vi "PC_Daten zu cRIO.vi"   [LabVIEW 2020, in "Kommunikation mit cRIO.lvlib"]
uses:
  Kommunikation mit cRIO.lvlib
  Bildwechsel/Bild-Auswahl.ctl
  Aktionen FGV Druckregler.ctl
  Funktionstasten/Funktionstasten-Aktion.ctl
  Seiten/Gaszuordnung AO/ANA-OUT Aktionen.ctl
  Seiten/Erweiterte Konfig/FGV PID Aktionen.ctl
  Stoerungen/FGV Stoerung aufnehmen Aktion.ctl
  Seiten/Erweiterte Konfig/Aktionen LN2 Dewar Spuelen.ctl
  EPA 1065/Dichtheitstest 1065-345/Aktion Leak Daten.ctl
  Funktionstasten/FGV Erweiterte Bedienung Aktion.ctl
  Seiten/CalGas Aufschaltung/FGV CalGas Aktionen.ctl
  Auto Kalibrieren/Aktion FGV CalZustand.ctl
  Status Analysatoren/Aktion Status Analysatoren.ctl
  Seiten/System Einstellungen V2/Aktioen FGV System.ctl
  Seiten/System Einstellungen V2/Aktioen FGV System Konstanten.ctl
  Auto Kalibrieren/Aktion FGV Autokal GT.ctl
  Seiten/Anlagengrenzwerte/Aktion Durchflussaenderung.ctl
  Allgemein/Aktion FGV Aufheizphase.ctl
  EPA 1065/T90 1065-308/Aktion FGV T90.ctl
  Seiten/Anlagenuebersicht/VisBx Anzeige/Aktion FGV Ventile manuell schalten Crio.ctl
  Allgemein/Aktionen Daten am cRIO speichern.ctl
  Seiten/Anlagengrenzwerte/FGV Anlagengrenzwerte Aktionen.ctl
  Seiten/CAN Konfig/Aktion FGV CAN.ctl
  Seiten/Anlagengrenzwerte/Anlagengrenzwerte.lvlib
  Seiten/Erweiterte Konfig/Erweiterte Konfig.lvlib
  Bildwechsel/Bildwechsel.lvlib
  Allgemein/allgemeine Sub-VIs.lvlib
  Funktionstasten/Funktionstasten.lvlib
  Seiten/Gaszuordnung AO/Gaszuordnung AO.lvlib
  Stoerungen/Stoerungen.lvlib
  Seiten/System Einstellungen V2/System Einstellungen V2.lvlib
  EPA 1065/Dichtheitstest 1065-345/Dichtheitstest 1065-345.lvlib
  Auto Kalibrieren/Auto Kalibrieren.lvlib
  Seiten/CalGas Aufschaltung/CalGas Aufschaltung.lvlib
  Status Analysatoren/Status Analysatoren.lvlib
  EPA 1065/T90 1065-308/T90 Test 1065-308.lvlib
  Seiten/Anlagenuebersicht/VisBx Anzeige/Anlagenuebersicht.lvlib
  Seiten/CAN Konfig/CAN Konfig.lvlib
types:
  T1 = typedef "Anlagenuebersicht.lvlib/Aktion FGV Ventile manuell schalten Crio.ctl" = enum16{"lesen", "Ventile schalten", "Testbetrieb aktiv", "Testbetrieb inaktiv", "Anzeige Ventilstellung"}
  T2 = typedef "EPA 1065.lvlib/T90 Test 1065-308.lvlib/Aktion FGV T90.ctl" = enum16{"lesen", "Konfig Daten", "speichern", "laden", "T90 aktiv", "T90 inaktiv", "Ext. Ventil aktivieren", "Ext. Ventil deaktivieren", "N2 spülen aktiv", "N2 spülen inaktiv", "Ergebnis Textfile"}
  T3 = typedef "allgemeine Sub-VIs.lvlib/Aktion FGV Aufheizphase.ctl" = enum16{"init", "lesen", "PNS Filterblock", "PNS HL1", "PNS HL2", "PNS HL3", "PNS HL4", "FTIR Messzelle", "HL 1", "HL 2", "HL zu FTIR", "auswerten"}
  T4 = typedef "Bildwechsel.lvlib/Bild-Auswahl.ctl" = enum16{"lesen", "Initialisieren", "Beenden", "Grafik", "Anlagenübersicht", "Anlagengrenzwerte", "Log Konfig", "Gaszuordnung AO", "Erw. Konfiguration", "FT-IR  ", "Störmeldungen", "Störmeldepuffer", "Störmeldekonfig", "PNS Grenzwerte", "Statusübersicht", "Linearisierung", "ARN", "EPA Dichtheitstest", "FID", "PMA", "CalGas", "Lambda", "Interference", "Amium PNS", "EPA T90", "Interference N2O", "Scheduler", "Systemeinstellungen", "EPA Drift", "CAN Konfig"}
  T5 = typedef "Anlagengrenzwerte.lvlib/Aktion Durchflussaenderung.ctl" = enum16{"lesen", "Statusänderung", "Reset"}
  T6 = typedef "Auto Kalibrieren.lvlib/Aktion FGV Autokal GT.ctl" = enum16{"lesen", "Autokal GT", "Referenz Start"}
  T7 = typedef "System Einstellungen V2.lvlib/Aktioen FGV System Konstanten.ctl" = enum16{"lesen", "laden", "speichern", "Sprache"}
  T8 = typedef "System Einstellungen V2.lvlib/Aktioen FGV System.ctl" = enum16{"lesen", "laden", "speichern", "Optionen schreiben", "Zeitstempel", "Reset BMP", "Reset SQP", "Wartung", "Werkseinstellung"}
  T9 = typedef "Status Analysatoren.lvlib/Aktion Status Analysatoren.ctl" = enum16{"lesen", "initialisieren", "Analysatoren aktiv", "FTIR Fehler", "FID Fehler", "PMA Fehler", "Felder einfärben"}
  T10 = typedef "Auto Kalibrieren.lvlib/Aktion FGV CalZustand.ctl" = enum16{"lesen", "Cal FTIR", "Cal FID CH4", "Cal PMA", "init", "Cal FID THC", "THC CG Eingang"}
  T11 = typedef "CalGas Aufschaltung.lvlib/FGV CalGas Aktionen.ctl" = enum16{"lesen", "Analysator Auswahl", "Def.CalGas", "Aufschaltung CalGas", "laden", "speichern", "KAL extrahieren"}
  T12 = typedef "Funktionstasten.lvlib/FGV Erweiterte Bedienung Aktion.ctl" = enum16{"Lesen", "Initialisieren", "N2 zu PNS", "Chart wechsel"}
  T13 = typedef "EPA 1065.lvlib/Dichtheitstest 1065-345.lvlib/Aktion Leak Daten.ctl" = enum16{"lesen", "laden", "speichern", "Volumen", "berechnen", "Leak check aktiv", "Leak Zustand", "Pfad", "Pfad speichern"}
  T14 = typedef "Erweiterte Konfig.lvlib/Aktionen LN2 Dewar Spuelen.ctl" = enum16{"lesen", "schreiben", "prüfen"}
  T15 = typedef "Stoerungen.lvlib/FGV Stoerung aufnehmen Aktion.ctl" = enum16{"Initialisieren", "Schreiben", "Lesen", "Quittieren", "quit. löschen"}
  T16 = typedef "Erweiterte Konfig.lvlib/FGV PID Aktionen.ctl" = enum16{"Lesen", "Schreiben PID", "Schreiben Sonstige", "Dichtheitstest", "Aktionen Dicht.", "Parameter Sensor"}
  T17 = typedef "Gaszuordnung AO.lvlib/ANA-OUT Aktionen.ctl" = enum16{"lesen", "Gase schreiben"}
  T18 = typedef "Funktionstasten.lvlib/Funktionstasten-Aktion.ctl" = enum16{"Initialisieren", "Zustand setzen", "Taste gedrückt", "Fehler speichern", "Lesen", "Manuell", "Remote", "Bitparallel", "Samplepoint", "Zeit Prüfen", "reset Umschalten"}
  T19 = typedef "Kommunikation mit cRIO.lvlib/Aktionen FGV Druckregler.ctl" = enum16{"lesen", "Parameter", "Istwerte", "laden", "speichern"}
  T20 = typedef "Status Analysatoren.lvlib/Status.ctl" = cluster{"FT-IR aktiv":bool, "FT-IR Fehler":bool, "FID aktiv":bool, "FID Fehler":bool, "PMA aktiv":bool, "PMA Fehler":bool}
  T21 = typedef "Erweiterte Konfig.lvlib/Aktionen Dichtheitstest.ctl" = enum16{"Initialisieren", "Unterdruck aufbauen", "Prop schließen", "Warten", "Auswertung", "Fertig"}
  T22 = typedef "System Einstellungen V2.lvlib/Optionen.ctl" = cluster{"Störmeldep.":bool, "Betriebszustände":bool, "AK in ppm":bool, "log Cal-Gas":bool, "log 0-Gas":bool, "Durchflusssensor 0-5V":bool, "PNS?":bool, "Mit N2 spülen":bool, "TRE08":bool, "Amium 10-Fach":bool, "Verticale Scrollbar aktiv":bool, "Loggingtakt":bool, "AK Rezeptwechsel gleich wie MKS":bool, "NG ECO":bool}
  T23 = typedef "EPA 1065.lvlib/Dichtheitstest 1065-345.lvlib/Aktion Leak check durchfuehren.ctl" = enum16{"initialisieren", "Unterdruck erzeugen", "Ventile schließen", "Warten", "Auswertung", "fertig", "PDF erstellen", "abbrechen"}
  T24 = typedef "CalGas Aufschaltung.lvlib/Aufschaltung CalGas.ctl" = cluster{"Kalibriergas":T25, "Aufschaltpunkt":T26, "Analysator":T27}
  T25 = typedef "Auswahlfeld.ctl" = u16
  T26 = typedef "CalGas Aufschaltung.lvlib/Auswahl Aufschaltpunkt.ctl" = enum16{"über Filterblock", "Analysator direkt", "über PNS", "Entnahme", "Gasdivider"}
  T27 = typedef "CalGas Aufschaltung.lvlib/Auswahl Analysator.ctl" = enum16{"FT-IR", "FID", "PMA", "PMA/FID/FT-IR"}
  T28 = typedef "allgemeine Sub-VIs.lvlib/Aktionen Daten am cRIO speichern.ctl" = enum16{"lesen", "speichern setzen", "speichern reset", "gespeichert"}
  T29 = typedef "Anlagengrenzwerte.lvlib/FGV Anlagengrenzwerte Aktionen.ctl" = enum16{"Lesen", "Grenzwerte schreiben"}
  T30 = typedef "CAN Konfig.lvlib/Aktion FGV CAN.ctl" = enum16{"lesen", "schreiben Konfig", "Status", "Messdaten", "laden", "speichern", "CAN Data"}
  T31 = typedef "Anlagengrenzwerte.lvlib/Anlagen-Grenzwerte Anzeige.ctl" = cluster{"Eingangsdruck FT-IR:":T32, "Durchfluss FT-IR:":T32, "Durchfluss CalGas:":T32, "Druck Ausgang:":T32, "Druck Kalter Block:":T32, "Heizleitungen intern:":T32, "Heizleitung zu FT-IR:":T32, "Heizung Filterblock:":T32, "Heizung Pumpe:":T32, "Heizleitung Extern SP1:":T32, "Heizleitung Extern SP2:":T32, "FT-IR Heizung Messzelle:":T32, "Schaltschranktemperatur:":T32, "Gaskühler:":T32}
  T32 = typedef "Anlagengrenzwerte.lvlib/Anlagen-Parameter Anzeige.ctl" = cluster{"Sollwert":sgl, "Warn-Min":sgl, "Warn-Max":sgl, "Abschalt-Min":sgl, "Abschalt-Max":sgl, "Regler":u16}
  T33 = cluster{"Sollwert":sgl, "Warn-Min":sgl, "Warn-Max":sgl, "Abschalt-Min":sgl, "Abschalt-Max":sgl, "Regler":sgl}
  T34 = typedef "Erweiterte Konfig.lvlib/Sonstige Parameter.ctl" = cluster{"Lüfter langsam":sgl, "Lüfter schnell":sgl, "FT-IR Kühlung Soll":sgl, "FT-IR Kühlung Max":sgl, "Überwachung":T25, "Befüllung aktiv":T35, "Stickstoff Befüllzeit":sgl, "Befüllintervall":sgl, "Kalibrierwert FT-IR":sgl, "Offset Ausgang":sgl, "Offset FT-IR":sgl, "Offset Druck FT-IR":sgl, "Dichtheitstest Zeit":sgl, "Dichtheitstest Abfall":sgl, "Dichtheitstest Umfang":T36, "Offset Umgebung":sgl, "Max Taupunkt":sgl, "Pumpendrehzahl":sgl, "ext. Befüllung":T35, "Ext. Stickstoff Befüllzeit":sgl}
  T35 = typedef "LogKonfig.lvlib/Auswahlfeld aktiviert-deaktiviert.ctl" = u16
  T36 = typedef "Erweiterte Konfig.lvlib/Dichtheitstest Umfang.ctl" = u16
  T37 = typedef "Erweiterte Konfig.lvlib/PID-Parameter Anzeige.ctl" = cluster{"Heizung\nFilterblock":T38, "Heizung\nPumpe":T38, "Heizung\nHeizleitungen":T38, "Heizleitung\nExtern":T38, "Heizung\nFB-Druckregler":T38}
  T38 = typedef "Erweiterte Konfig.lvlib/PID-Parameter.ctl" = cluster{"P-Anteil":T39, "I-Anteil":T39, "D-Anteil":T39, "Regelzonengr.":T39, "max. OUT":T39}
  T39 = typedef "Zahlen-Eingabefeld.ctl" = sgl
  T40 = typedef "Erweiterte Konfig.lvlib/Parameter Sensoren.ctl" = cluster{"Kal.Durchfl.FTIR":sgl, "Kal.Durchfl.PMA":sgl, "Offset Durchfl.FTIR":sgl, "Offset Druck Ausgang":sgl, "Offset Druck Umgebung":sgl, "Offset Durchfl.PMA":sgl, "Offset Druck CG PMA":sgl, "Offset Druck CG":sgl, "Offset Druck FTIR IAG":sgl, "Druck Kalter Block":sgl}
  T41 = cluster{"Lüfter langsam":sgl, "Lüfter schnell":sgl, "FT-IR Kühlung Soll":sgl, "FT-IR Kühlung Max":sgl, sgl, sgl, "Stickstoff Befüllzeit":sgl, "Befüllintervall":sgl, "Kalibrierwert FT-IR":sgl, "Offset Ausgang":sgl, "Offset FT-IR":sgl, "Offset Druck FT-IR":sgl, "Dichtheitstest Zeit":sgl, "Dichtheitstest Abfall":sgl, sgl, "Offset Umgebung":sgl, "Max Taupunkt":sgl, "Pumpendrehzahl":sgl, sgl, "Ext. Stickstoff Befüllzeit":sgl}
  T42 = typedef "CAN Konfig.lvlib/Konfig Daten PC.ctl" = cluster{"Baude Rate":T43, "COM state":u8, "Frame-ID FTIR Start":u32, "Frame-ID FTIR End":u32, "Frame-ID Status Start":u32, "Frame-ID Status End":u32, "Zustand Information":u32, "Aktion":u32, "Frame-ID FTIR Arry":u32[], "Frame-ID Status Arry":u32[], "GPS Start":u32, "Interface":refnum<k21>}
  T43 = typedef "CAN Interface.lvlib/Baude Rate.ctl" = u32
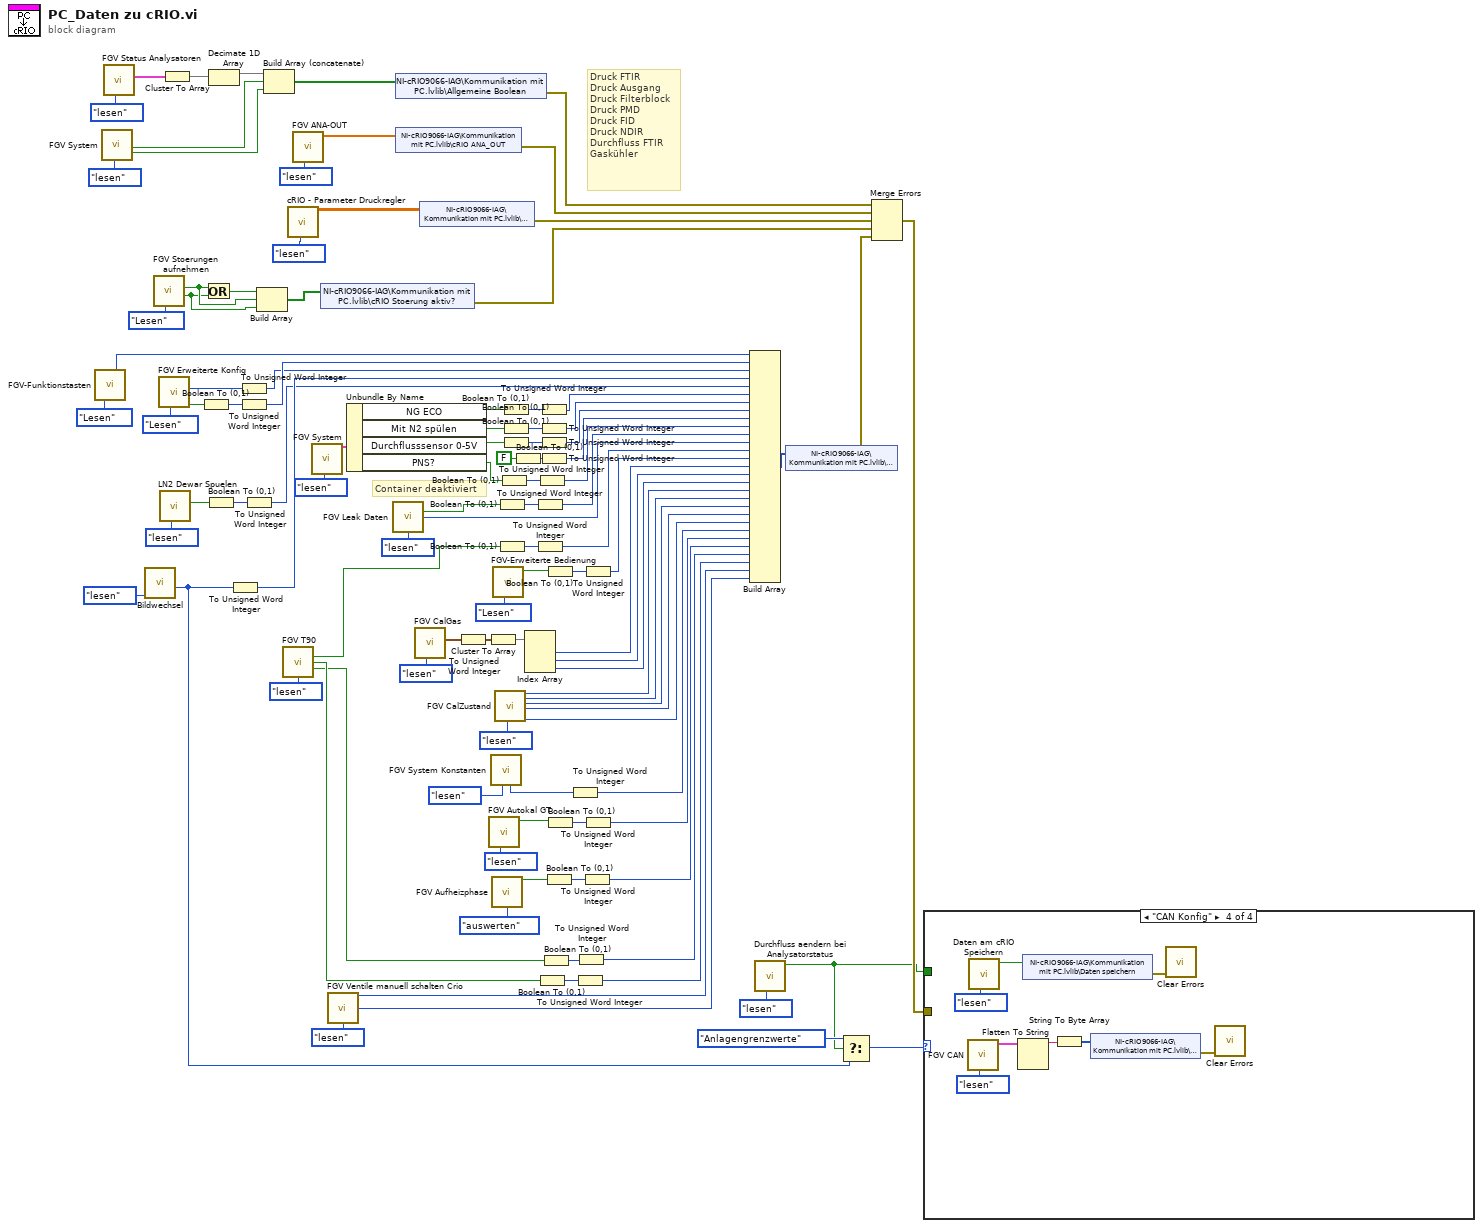
[diagram p0: block diagram]
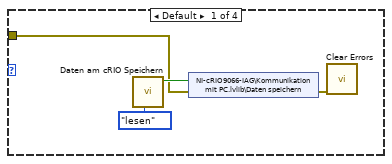
[diagram p2: hidden frame]
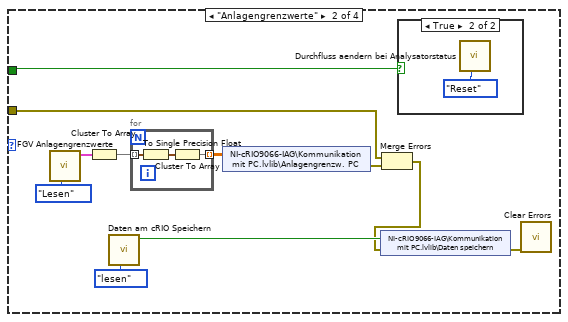
[diagram p3: hidden frame]
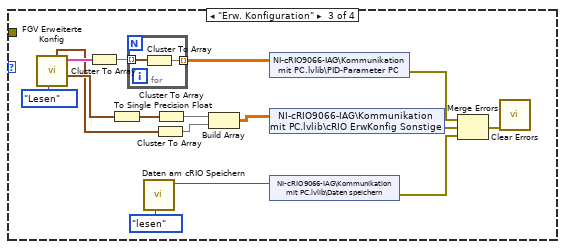
[diagram p5: hidden frame]
diagram:
  # "Container deaktiviert"
  # "Druck FTIR\nDruck Ausgang\nDruck Filterblock\nDruck PMD\nDruck FID\nDruck NDIR\nDurchfluss FTIR\nGaskühler"
  n1 = call "FGV-Funktionstasten.vi"("Aktion"=Funktionstasten-Aktion."Lesen") -> ("Samplepoint"=w101:u16)  [unwired: 7 in, 7 out]
  n2 = call "FGV System.vi"("Aktionen"=Aktioen_FGV_System."lesen") -> ("Reset BMP"=w36:bool, "Reset SQP"=w35:bool)  [unwired: 12 in, 5 out]
  n3 = call "FGV Status Analysatoren.vi"("Aktionen"=Aktion_Status_Analysatoren."lesen") -> ("Status Analysatoren"=w41:T20)  [unwired: 10 in]
  n4 = call "Bildwechsel.vi"("nächstes Bild"=Bild-Auswahl."lesen") -> ("aktuelle Bildnummer"=w23:T4)  [unwired: 9 in, 1 out]
  n5 = call "FGV Stoerungen aufnehmen.vi"("FGV Störung aufnehmen Aktion"=FGV_Stoerung_aufnehmen_Aktion."Lesen") -> ("abschalten"=w14:bool, "warnen"=w15:bool)  [unwired: 7 in, 2 out]
  n6 = call "FGV Erweiterte Konfig.vi"("Aktion"=FGV_PID_Aktionen."Lesen") -> ("Dichtheitstest?"=w98:bool, "Aktionen Dichtheitstest"=w99:T21)  [unwired: 6 in, 3 out]
  n7 = call "LN2 Dewar Spuelen.vi"("Aktionen"=Aktionen_LN2_Dewar_Spuelen."lesen") -> ("LN2 Spülen?"=w83:bool)  [unwired: 10 in]
  n8 = Cluster To Array(cluster=w41) -> (array=w40:bool[])
  n9 = Boolean To (0,1)(Boolean=w98) -> (0, 1=w100:i16)
  n10 = Or(x=w15, y=w14) -> (x .or. y?=w86:bool)
  n11 = Boolean To (0,1)(Boolean=w83) -> (0, 1=w84:i16)
  n12 = Decimate 1D Array(w40) -> (w39:bool[])  [unwired: 1 out]
  n13 = To Unsigned Word Integer(number=w23) -> (unsigned 16bit integer=w95:u16)
  n14 = To Unsigned Word Integer(number=w99) -> (unsigned 16bit integer=w96:u16)
  n15 = To Unsigned Word Integer(number=w100) -> (unsigned 16bit integer=w97:u16)
  n16 = To Unsigned Word Integer(number=w84) -> (unsigned 16bit integer=w82:u16)
  n17 = Build Array(w86, w15, w14) -> (w16:bool[])
  n18 = Build Array (concatenate)(w39, w36, w35) -> (w38:bool[])
  n19 = call "FGV T90.vi"("Aktion"=Aktion_FGV_T90."lesen") -> ("T90 Aktiv"=w10:bool, "Ext. Ventil aktiv"=w8:bool, "N2 spülen aktiv"=w7:bool)  [unwired: 9 in, 3 out]
  n20 = call "cRIO - Parameter Druckregler.vi"("Aktion"=Aktionen_FGV_Druckregler."lesen") -> ("Parameter Regler"=w93:sgl[][])  [unwired: 9 in, 9 out]
  n21 = call "FGV ANA-OUT.vi"("Aktion"=ANA-OUT_Aktionen."lesen") -> ("ANA-OUT 1-16"=w91:sgl[])  [unwired: 10 in]
  n22 = call "FGV System.vi"("Aktionen"=Aktioen_FGV_System."lesen") -> ("Optionen"=w80:T22)  [unwired: 12 in, 6 out]
  n23 = shared-variable "NI-cRIO9066-IAG\\Kommunikation mit PC.lvlib\\cRIO Stoerung aktiv?"(w16) -> (error out=w94:errorcluster)  [unwired: 1 in]
  n24 = call "FGV Ventile manuell schalten Crio.vi"("Aktion"=Aktion_FGV_Ventile_manuell_schalten_Crio."lesen") -> ("Ventile schalten"=w2:u32, "Betrieb"=w1:u16)  [unwired: 11 in, 2 out]
  n25 = Unbundle By Name(w80) -> ("NG ECO"=w4:bool, "Mit N2 spülen"=w76:bool, "Durchflusssensor 0-5V"=w73:bool, "PNS?"=w69:bool)
  n26 = call "FGV Leak Daten.vi"("Aktion"=Aktion_Leak_Daten."lesen") -> ("Dichtheitstest aktiv"=w65:bool, "Dichtheitstest Zustand"=w63:T23)  [unwired: 10 in, 3 out]
  n27 = shared-variable "NI-cRIO9066-IAG\\Kommunikation mit PC.lvlib\\Allgemeine Boolean"(w38) -> (error out=w43:errorcluster)  [unwired: 1 in]
  n28 = shared-variable "NI-cRIO9066-IAG\\Kommunikation mit PC.lvlib\\cRIO ANA_OUT"(w91) -> (error out=w90:errorcluster)  [unwired: 1 in]
  n29 = call "FGV CalGas.vi"("Aktionen"=FGV_CalGas_Aktionen."lesen") -> ("Aufschaltung CalGas"=w53:T24)  [unwired: 6 in, 4 out]
  n30 = shared-variable "NI-cRIO9066-IAG\\Kommunikation mit PC.lvlib\\Param.Regler"(w93) -> (error out=w92:errorcluster)  [unwired: 1 in]
  n31 = To Unsigned Word Integer(number=w53) -> (unsigned 16bit integer=w52:cluster{"Kalibriergas":T25, u16, u16})
  n32 = Cluster To Array(cluster=w52) -> (array=w51:T25[])
  n33 = call "FGV Autokal GT.vi"("Aktion FGV AutoKal"=Aktion_FGV_Autokal_GT."lesen") -> ("Autokal GT Aktiv?"=w28:bool)  [unwired: 8 in, 2 out]
  n34 = call "FGV System Konstanten.vi"("Aktionen"=Aktioen_FGV_System_Konstanten."lesen") -> ("SysLogLevel"=w32:u32)  [unwired: 6 in, 4 out]
  n35 = call "FGV Aufheizphase.vi"("Aktion"=Aktion_FGV_Aufheizphase."auswerten") -> ("Aufheizphase"=w18:bool)  [unwired: 12 in, 2 out]
  n36 = call "FGV-Erweiterte Bedienung.vi"("Aktion"=FGV_Erweiterte_Bedienung_Aktion."Lesen") -> ("N2 zu PNS"=w57:bool)  [unwired: 9 in, 1 out]
  n37 = call "FGV CalZustand.vi"("Aktion"=Aktion_FGV_CalZustand."lesen") -> ("CAL Zustand FTIR"=w47:u16, "CAL Zustand PMA"=w46:u16, "CAL Zustand FID CH4"=w45:u16, "CAL Zustand FID THC"=w44:u16, "CG Eingang"=w34:u16)  [unwired: 14 in]
  n38 = Boolean To (0,1)(Boolean=w65) -> (0, 1=w66:i16)
  n39 = Boolean To (0,1)(Boolean=w10) -> (0, 1=w61:i16)
  n40 = Boolean To (0,1)(Boolean=w69) -> (0, 1=w68:i16)
  n41 = Boolean To (0,1)(Boolean=w4) -> (0, 1=w79:i16)
  n42 = Boolean To (0,1)(Boolean=w76) -> (0, 1=w77:i16)
  n43 = Boolean To (0,1)(Boolean=w73) -> (0, 1=w74:i16)
  n44 = Boolean To (0,1)(Boolean=FALSE ("Reserve-Container")) -> (0, 1=w71:i16)
  n45 = Index Array(array=w51) -> (element #1=w50:T25, element #2=w49:T25, element #3=w48:T25)  [unwired: 3 in]
  n46 = To Unsigned Word Integer(number=w66) -> (unsigned 16bit integer=w64:u16)
  n47 = To Unsigned Word Integer(number=w61) -> (unsigned 16bit integer=w60:u16)
  n48 = To Unsigned Word Integer(number=w68) -> (unsigned 16bit integer=w67:u16)
  n49 = Boolean To (0,1)(Boolean=w8) -> (0, 1=w9:i16)
  n50 = To Unsigned Word Integer(number=w79) -> (unsigned 16bit integer=w78:u16)
  n51 = To Unsigned Word Integer(number=w77) -> (unsigned 16bit integer=w75:u16)
  n52 = To Unsigned Word Integer(number=w74) -> (unsigned 16bit integer=w72:u16)
  n53 = To Unsigned Word Integer(number=w71) -> (unsigned 16bit integer=w70:u16)
  n54 = Boolean To (0,1)(Boolean=w7) -> (0, 1=w6:i16)
  n55 = Boolean To (0,1)(Boolean=w18) -> (0, 1=w19:i16)
  n56 = Boolean To (0,1)(Boolean=w57) -> (0, 1=w58:i16)
  n57 = Boolean To (0,1)(Boolean=w28) -> (0, 1=w29:i16)
  n58 = To Unsigned Word Integer(number=w32) -> (unsigned 16bit integer=w31:u16)
  n59 = To Unsigned Word Integer(number=w9) -> (unsigned 16bit integer=w12:u16)
  n60 = To Unsigned Word Integer(number=w6) -> (unsigned 16bit integer=w13:u16)
  n61 = To Unsigned Word Integer(number=w19) -> (unsigned 16bit integer=w17:u16)
  n62 = To Unsigned Word Integer(number=w58) -> (unsigned 16bit integer=w56:u16)
  n63 = To Unsigned Word Integer(number=w29) -> (unsigned 16bit integer=w27:u16)
  n64 = Build Array(w101, w97, w96, w95, w82, w78, w75, w72, w70, w67, w64, w63, w60, w56, w50, w49, w48, w47, w46, w45, w44, w34, w31, w27, w17, w13, w12, w2, w1) -> (w89:u32[])
  n65 = call "Durchfluss aendern bei Analysatorstatus.vi"("Aktion"=Aktion_Durchflussaenderung."lesen") -> ("Durchflussänderung"=w21:bool)  [unwired: 9 in, 1 out]
  n66 = shared-variable "NI-cRIO9066-IAG\\Kommunikation mit PC.lvlib\\Samplepoint"(w89) -> (error out=w88:errorcluster)  [unwired: 1 in]
  n67 = Select(t=Bild-Auswahl."Anlagengrenzwerte", s=w21, f=w23) -> (s? t:f=w24:T4)
  n68 = Merge Errors(w43, w90, w92, w94, w88) -> (w26:errorcluster)
  n69 = case shown="\"CAN Konfig\"" w24 {
    tunnel: w26 -> [w107 w114 _ _]
    tunnel: w21 -> [_ w111 _ _]
    frame Default {
      n70 = call "Daten am cRIO Speichern.vi"("Aktionen"=Aktionen_Daten_am_cRIO_speichern."lesen") -> ("speichern"=w109:bool)  [unwired: 9 in, 1 out]
      n71 = shared-variable "NI-cRIO9066-IAG\\Kommunikation mit PC.lvlib\\Daten speichern"(w109, error in=w107) -> (error out=w108:errorcluster)
      n72 = call <vilib>:"Clear Errors.vi"("error in (no error)"=w108) -> ()  [unwired: 5 in, 2 out]
    }
    frame "Anlagengrenzwerte" {
      n73 = call "FGV Anlagengrenzwerte.vi"("Aktion"=FGV_Anlagengrenzwerte_Aktionen."Lesen") -> ("Anlagen-Grenzwerte Anzeige"=w118:T31)  [unwired: 10 in]
      n74 = Cluster To Array(cluster=w118) -> (array=w119:T32[])
      n75 = call "Daten am cRIO Speichern.vi"("Aktionen"=Aktionen_Daten_am_cRIO_speichern."lesen") -> ("speichern"=w117:bool)  [unwired: 9 in, 1 out]
      n76 = for {
        tunnel: w119 -> [w125] mode=indexing
        tunnel: [w123] -> w115 mode=indexing
        n77 = To Single Precision Float(number=w125) -> (single precision float=w124:T33)
        n78 = Cluster To Array(cluster=w124) -> (array=w123:sgl[])
      }
      n79 = shared-variable "NI-cRIO9066-IAG\\Kommunikation mit PC.lvlib\\Anlagengrenzw. PC"(w115) -> (error out=w116:errorcluster)  [unwired: 1 in]
      n80 = Merge Errors(w114, w116) -> (w113:errorcluster)
      n81 = shared-variable "NI-cRIO9066-IAG\\Kommunikation mit PC.lvlib\\Daten speichern"(w117, error in=w113) -> (error out=w112:errorcluster)
      n82 = case shown="True" w111 {
        frame False {
        }
        frame True {
          n83 = call "Durchfluss aendern bei Analysatorstatus.vi"("Aktion"=Aktion_Durchflussaenderung."Reset") -> ()  [unwired: 9 in, 2 out]
        }
      }
      n84 = call <vilib>:"Clear Errors.vi"("error in (no error)"=w112) -> ()  [unwired: 5 in, 2 out]
    }
    frame "Erw. Konfiguration" {
      n85 = call "FGV Erweiterte Konfig.vi"("Aktion"=FGV_PID_Aktionen."Lesen") -> ("Sonstige"=w137:T34, "PID-Parameter Anzeige"=w138:T37, "Parameter Sensoren"=w127:T40)  [unwired: 5 in, 3 out]
      n86 = Cluster To Array(cluster=w138) -> (array=w139:T38[])
      n87 = To Single Precision Float(number=w137) -> (single precision float=w129:T41)
      n88 = for {
        tunnel: w139 -> [w143] mode=indexing
        tunnel: [w142] -> w135 mode=indexing
        n89 = Cluster To Array(cluster=w143) -> (array=w142:T39[])
      }
      n90 = call "Daten am cRIO Speichern.vi"("Aktionen"=Aktionen_Daten_am_cRIO_speichern."lesen") -> ("speichern"=w134:bool)  [unwired: 9 in, 1 out]
      n91 = Cluster To Array(cluster=w127) -> (array=w128:sgl[])
      n92 = Cluster To Array(cluster=w129) -> (array=w130:sgl[])
      n93 = Build Array(w130, w128) -> (w126:sgl[][])
      n94 = shared-variable "NI-cRIO9066-IAG\\Kommunikation mit PC.lvlib\\PID-Parameter PC"(w135) -> (error out=w133:errorcluster)  [unwired: 1 in]
      n95 = shared-variable "NI-cRIO9066-IAG\\Kommunikation mit PC.lvlib\\cRIO ErwKonfig Sonstige"(w126) -> (error out=w132:errorcluster)  [unwired: 1 in]
      n96 = shared-variable "NI-cRIO9066-IAG\\Kommunikation mit PC.lvlib\\Daten speichern"(w134) -> (error out=w131:errorcluster)  [unwired: 1 in]
      n97 = Merge Errors(w133, w132, w131) -> (w136:errorcluster)
      n98 = call <vilib>:"Clear Errors.vi"("error in (no error)"=w136) -> ()  [unwired: 5 in, 2 out]
    }
    frame "CAN Konfig" {
      n99 = call "FGV CAN.vi"("Aktion"=Aktion_FGV_CAN."lesen") -> ("Konfig Daten"=w146:T42)  [unwired: 6 in, 4 out]
      n100 = call "Daten am cRIO Speichern.vi"("Aktionen"=Aktionen_Daten_am_cRIO_speichern."lesen") -> ("speichern"=w150:bool)  [unwired: 9 in, 1 out]
      n101 = Flatten To String(anything=w146) -> (data string=w147:string)  [unwired: 3 in, 2 out]
      n102 = shared-variable "NI-cRIO9066-IAG\\Kommunikation mit PC.lvlib\\Daten speichern"(w150) -> (error out=w149:errorcluster)  [unwired: 1 in]
      n103 = String To Byte Array(string=w147) -> (unsigned byte array=w145:u8[])
      n104 = shared-variable "NI-cRIO9066-IAG\\Kommunikation mit PC.lvlib\\CAN_Konfig"(w145) -> (error out=w144:errorcluster)  [unwired: 1 in]
      n105 = call <vilib>:"Clear Errors.vi"("error in (no error)"=w149) -> ()  [unwired: 5 in, 2 out]
      n106 = call <vilib>:"Clear Errors.vi"("error in (no error)"=w144) -> ()  [unwired: 5 in, 2 out]
    }
  }
